vi "convertPhysicalChannelNames.vi"(8 "error in (no error)":errorcluster, 10 "PhysicalChannels":string, 11 "niDAQmxDO in":refnum<class "niDAQmxDO.lvclass">) -> (0 "error out":errorcluster, 2 "channel_names":string, 3 "niDAQmxDO out":refnum<class "niDAQmxDO.lvclass">)   [LabVIEW 2009, in "Hardware.lvlib" / "Channels.lvlib" / "niDAQmxDO.lvclass"]
uses:
  niDAQmxDO.lvclass
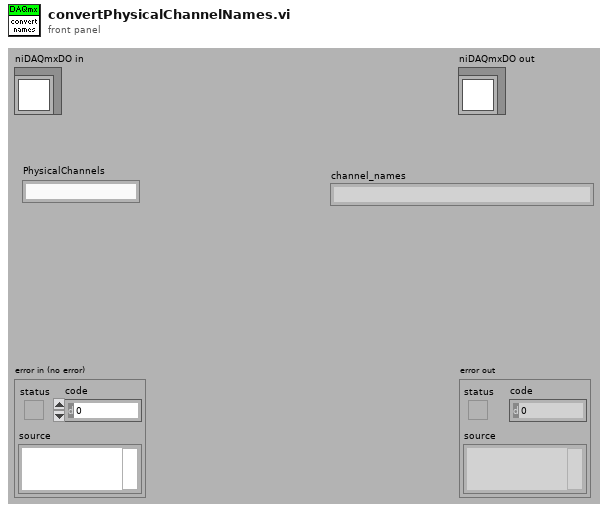
[diagram p1: front panel]
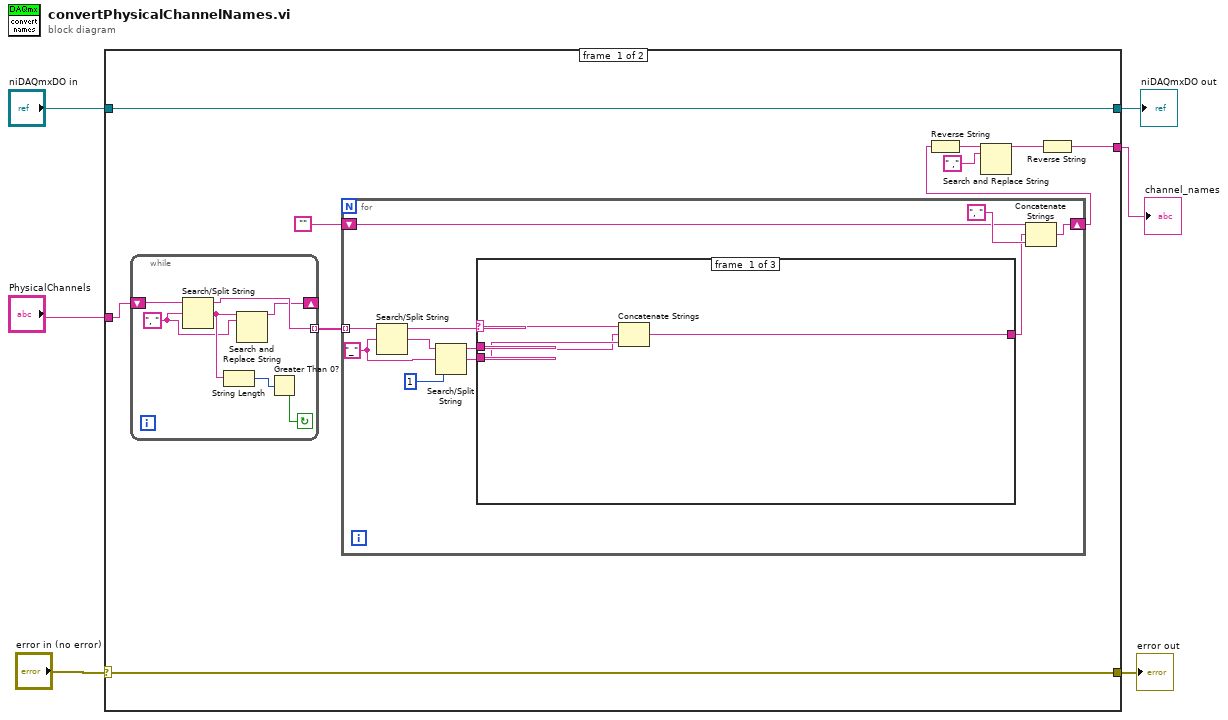
[diagram p0: block diagram]
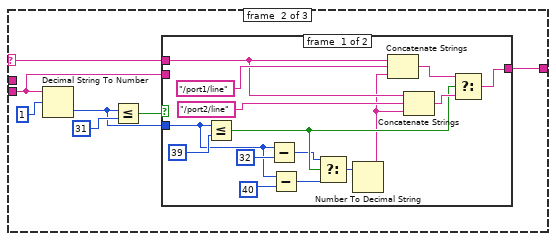
[diagram p2: hidden frame]
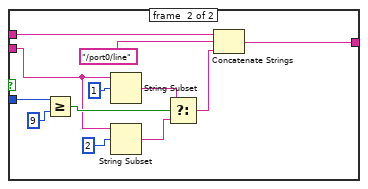
[diagram p3: hidden frame]
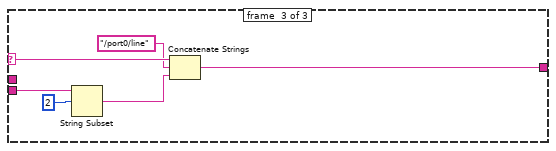
[diagram p4: hidden frame]
diagram:
  n1 = case shown="No Error" "error in (no error)" {
    selector: "error in (no error)" -> [w15 w80]
    tunnel: [w15 w80] -> w5
    tunnel: [w16 w79] -> w3
    tunnel: "niDAQmxDO in" -> [w16 w79]
    tunnel: "PhysicalChannels" -> [w14 _]
    tunnel: [w7 _] -> w1
    frame #0 {
      n2 = while {
        shift-right: [w74] -> _
        shift-left: w14 -> [w78]
        tunnel: [w77] -> w13 mode=indexing
        stop <- w72 continue-if-true
        w75 = ", "
        n3 = Search/Split String(string=w78, search string/char (-)=w75) -> (substring before match=w77:string, match + rest of string=w76:string)  [unwired: 1 in, 1 out]
        n4 = String Length(string=w76) -> (length=w73:i32)
        n5 = Search and Replace String(input string=w76, search string=w75) -> (result string=w74:string)  [unwired: 6 in, 3 out]
        n6 = Greater Than 0?(x=w73) -> (x > 0?=w72:bool)
      }
      n7 = for {
        tunnel: w13 -> [w21] mode=indexing
        shift-right: [w18] -> w8
        shift-left: "" -> [w19]
        w25 = "_"
        n8 = Search/Split String(string=w21, search string/char (-)=w25) -> (substring before match=w27:string, match + rest of string=w26:string)  [unwired: 1 in, 1 out]
        n9 = Search/Split String(string=w26, search string/char (-)=w25, offset (0)=1) -> (substring before match=w22:string, match + rest of string=w23:string)  [unwired: 1 out]
        n10 = case shown="\"DAQ\", \"UsbDAQ\"" w27 {
          selector: w27 -> [w31 w35 w69]
          tunnel: w23 -> [w29 w36 w71]
          tunnel: [w30 w33 w68] -> w17
          tunnel: w22 -> [w28 _ _]
          frame #0 {
            n11 = Concatenate Strings(w31, w28, w29) -> (w30:string)
          }
          frame #1 {
            n12 = Decimal String To Number(string=w36, offset=1) -> (number=w34:i32)  [unwired: 1 in, 1 out]
            n13 = Less Or Equal?(x=w34, y=31) -> (x <= y?=w37:bool)
            n14 = case shown="True" w37 {
              tunnel: w36 -> [_ w54]
              tunnel: w35 -> [w50 w65]
              tunnel: [w47 w63] -> w33
              tunnel: w34 -> [w45 w62]
              frame #0 {
                n15 = Less Or Equal?(x=w45, y=39) -> (x <= y?=w44:bool)
                n16 = Subtract(x=w45, y=32) -> (x-y=w43:i32)
                n17 = Subtract(x=w45, y=40) -> (x-y=w41:i32)
                n18 = Select(t=w43, s=w44, f=w41) -> (s? t:f=w40:i32)
                n19 = Number To Decimal String(number=w40) -> (decimal integer string=w39:string)  [unwired: 1 in]
                n20 = Concatenate Strings(w50, "/port1/line", w39) -> (w51:string)
                n21 = Concatenate Strings(w50, "/port2/line", w39) -> (w48:string)
                n22 = Select(t=w51, s=w44, f=w48) -> (s? t:f=w47:string)
              }
              frame #1 {
                n23 = Greater Or Equal?(x=w62, y=9) -> (x >= y?=w57:bool)
                n24 = String Subset(string=w54, offset (0)=1) -> (substring=w59:string)  [unwired: 1 in]
                n25 = String Subset(string=w54, offset (0)=2) -> (substring=w56:string)  [unwired: 1 in]
                n26 = Select(t=w59, s=w57, f=w56) -> (s? t:f=w55:string)
                n27 = Concatenate Strings(w65, "/port0/line", w55) -> (w63:string)
              }
            }
          }
          frame #2 {
            n28 = String Subset(string=w71, offset (0)=2) -> (substring=w66:string)  [unwired: 1 in]
            n29 = Concatenate Strings(w69, "/port0/line", w66) -> (w68:string)
          }
        }
        n30 = Concatenate Strings(w19, w17, ", ") -> (w18:string)
      }
      n31 = Reverse String(1:w8) -> (0:w11:string)
      n32 = Search and Replace String(input string=w11, search string=" ,") -> (result string=w9:string)  [unwired: 6 in, 3 out]
      n33 = Reverse String(1:w9) -> (0:w7:string)
    }
    frame #1 {
    }
  }
  "error out" <- w5
  "niDAQmxDO out" <- w3
  "channel_names" <- w1
